vi "prepareNonVegMeal.vi"(8 "error in (no error)":errorcluster, 11 "MealBuilder in":refnum<class "MealBuilder.lvclass">) -> (0 "error out":errorcluster, 2 "Meal out":refnum<class "Meal.lvclass">, 3 "MealBuilder out":refnum<class "MealBuilder.lvclass">)   [LabVIEW 2016, in "MealBuilder.lvclass"]
uses:
  MealBuilder.lvclass
  Meal Class/Meal.lvclass
  ChickenBurger Class/ChickenBurger.lvclass
  C:/Users/Felipe/Desktop/LabVIEW OOP Design Patters Folder/LabVIEW OOP Design Patters Folder/Builder Pattern/Item Class/Item.lvclass
  Pepsi Class/Pepsi.lvclass
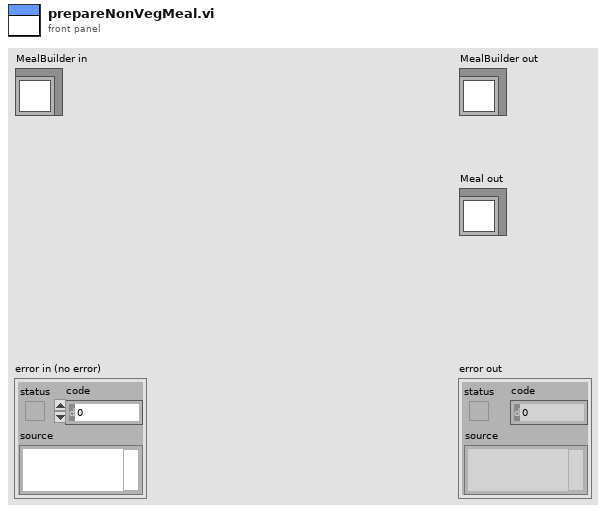
[diagram p1: front panel]
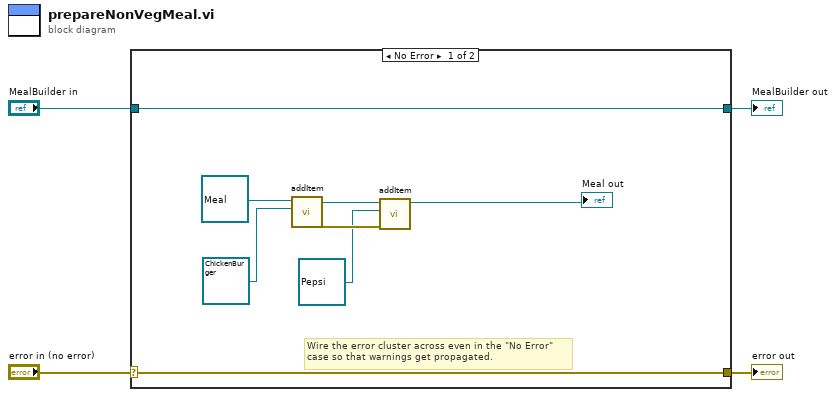
[diagram p0: block diagram]
diagram:
  n1 = case shown="No Error" "error in (no error)" {
    selector: "error in (no error)" -> [w11 w14]
    tunnel: [w11 w14] -> w3
    tunnel: [w12 w13] -> w1
    tunnel: "MealBuilder in" -> [w12 w13]
    frame No Error {
      # "Wire the error cluster across even in the \"No Error\"\ncase so that warnings get propagated."
      n2 = call-dynamic "addItem.vi"("Item.lvclass"=refnum<class "ChickenBurger.lvclass"> refnum ("ChickenBurger.lvclass"), "Meal in"=refnum<class "Meal.lvclass"> refnum ("Meal.lvclass")) -> ("error out"=w9:errorcluster, "Meal out"=w10:refnum<class "Meal.lvclass">)  [unwired: 8 in]
      n3 = call-dynamic "addItem.vi"("error in (no error)"=w9, "Item.lvclass"=refnum<class "Pepsi.lvclass"> refnum ("Pepsi.lvclass"), "Meal in"=w10) -> ("Meal out"=→"Meal out":refnum<class "Meal.lvclass">)  [unwired: 7 in, 1 out]
    }
    frame Error {
    }
  }
  "error out" <- w3
  "MealBuilder out" <- w1
